vi "Create Default System Config.vi"(8 "error in (no error)":errorcluster, 10 "System Config Path":path, 11 "App in":refnum<class "App.lvclass">) -> (0 "error out":errorcluster, 3 "App out":refnum<class "App.lvclass">)   [LabVIEW 2020, in "PicoG-App.lvlib" / "App.lvclass"]
uses:
  App.lvclass
  <vilib>/Utility/config.llb/NI_LVConfig.lvlib
  <vilib>/Utility/config.llb/Write Key (I32).vi
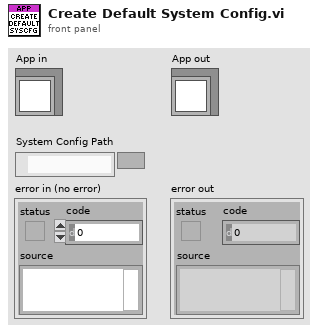
[diagram p1: front panel]
types:
  T1 = typedef "NI_LVConfig.lvlib/Config Data RefNum.ctl" = refnum<k1>
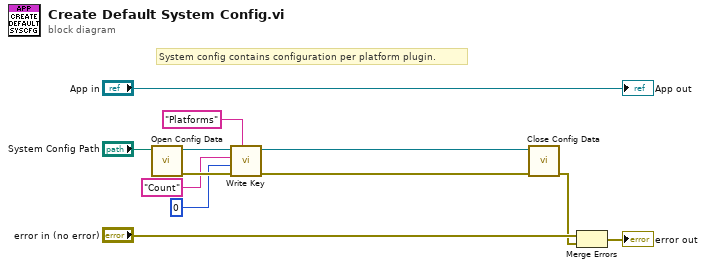
[diagram p0: block diagram]
diagram:
  # "System config contains configuration per platform plugin."
  n1 = call <vilib>:"Open Config Data.vi"("configuration file path"="System Config Path") -> ("error out"=w12:errorcluster, "refnum"=w8:T1)  [unwired: 8 in, 1 out]
  n2 = call-poly <vilib>:"Write Key.vi"("section"="Platforms", "error in (no error)"=w12, "value"=0, "key"="Count", "refnum"=w8) -> ("error out"=w3:errorcluster, "refnum out"=w4:T1)  [unwired: 4 in, 1 out]
  n3 = call <vilib>:"Close Config Data.vi"("error in (no error)"=w3, "refnum"=w4) -> ("error out"=w1:errorcluster)  [unwired: 8 in, 1 out]
  n4 = Merge Errors("error in (no error)", w1) -> (→"error out":errorcluster)
  "App out" <- "App in"
